vi "Rasnik_save.vi"() -> ()   [LabVIEW 2015]
uses:
  GlobalPath.vi
  Desktop/Mari/GlobalData.vi
panel:
  out "Script":path
  out "Logfile Path":path
  out "Filename selected":path
  out "standard output":string
  out "Y D10":dbl format="%.2f"
  out "Y D9":dbl format="%.2f"
  out "Y D8":dbl format="%.2f"
  out "Y D7":dbl format="%.2f"
  out "Y D6":dbl format="%.2f"
  out "Y D5":dbl format="%.2f"
  out "Y D4":dbl format="%.2f"
  out "Y D3":dbl format="%.2f"
  out "Y D2":dbl format="%.2f"
  out "Y D1":dbl format="%.2f"
  out "X D10":dbl format="%.2f"
  out "X D9":dbl format="%.2f"
  out "X D8":dbl format="%.2f"
  out "X D7":dbl format="%.2f"
  out "X D6":dbl format="%.2f"
  out "X D5":dbl format="%.2f"
  out "X D4":dbl format="%.2f"
  out "X D3":dbl format="%.2f"
  out "X D2":dbl format="%.2f"
  out "X D1":dbl format="%.2f"
  out "Latest file: 2":path
  out "y 6":string
  out "x 6":string
  in  "Done?":bool
  out "y 10":string
  out "x 10":string
  out "y 9":string
  out "x 9":string
  out "y 8":string
  out "x 8":string
  out "y 7":string
  out "x 7":string
  out "y 5":string
  out "x 5":string
  out "y 4":string
  out "x 4":string
  out "y 3":string
  out "x 3":string
  out "y 2":string
  out "x 2":string
  out "y 1":string
  out "x 1":string
  out "Lines":string[](array[string])
  out "Latest file:":path
  in  "Open Program":bool
  in  "c-ccd 3":bool caption="Setup the electronics for the C-CCD reading:\n- make sure the ethernet cables are connected on the minimal heads\n- check that the cable connecting the driver with the mux is plugged in\n- verify that the driver is on and connected to the LAN"
  in  "c-ccd":bool caption="Read the data file"
  # "Rasmask reading from PCBs on stiffback/table"
  # "Run the C-CCD reading program \n(the 10 Rasmasks are automatically read and the data saved)"
  # "Data file reading"
  # "The most recent data file created by the C-CCD program will be opened.\nOnce the \"read data file\" is clicked, the raw data and displacement should appear on the PCB schematics on the bottom."
  # "Displacement (um):"
  # "Raw Data (um):"
  # "Rasmask 1"
  # "Rasmask 2"
  # "Rasmask 1"
  # "Rasmask 2"
  # "Rasmask 3"
  # "Rasmask 4"
  # "Rasmask 3"
  # "Rasmask 4"
  # "Rasmask 6"
  # "Rasmask 5"
  # "Rasmask 6"
  # "Rasmask 5"
  # "Rasmask 7"
  # "Rasmask 8"
  # "Rasmask 7"
  # "Rasmask 8"
  # "Rasmask 9"
  # "Rasmask 10"
  # "Rasmask 9"
  # "Rasmask 10"
  # "Open the DB and load the Rarnik raw file:\nClick on the tab \"RO measurement\" and on the bottom click on \"Load Rasnik 1\" for the table and \"Load  Rasnik 2\" for the stiffback\nLoad the file that appears here --------------------------------------------------------------->\nPress \"SAve info to database\""
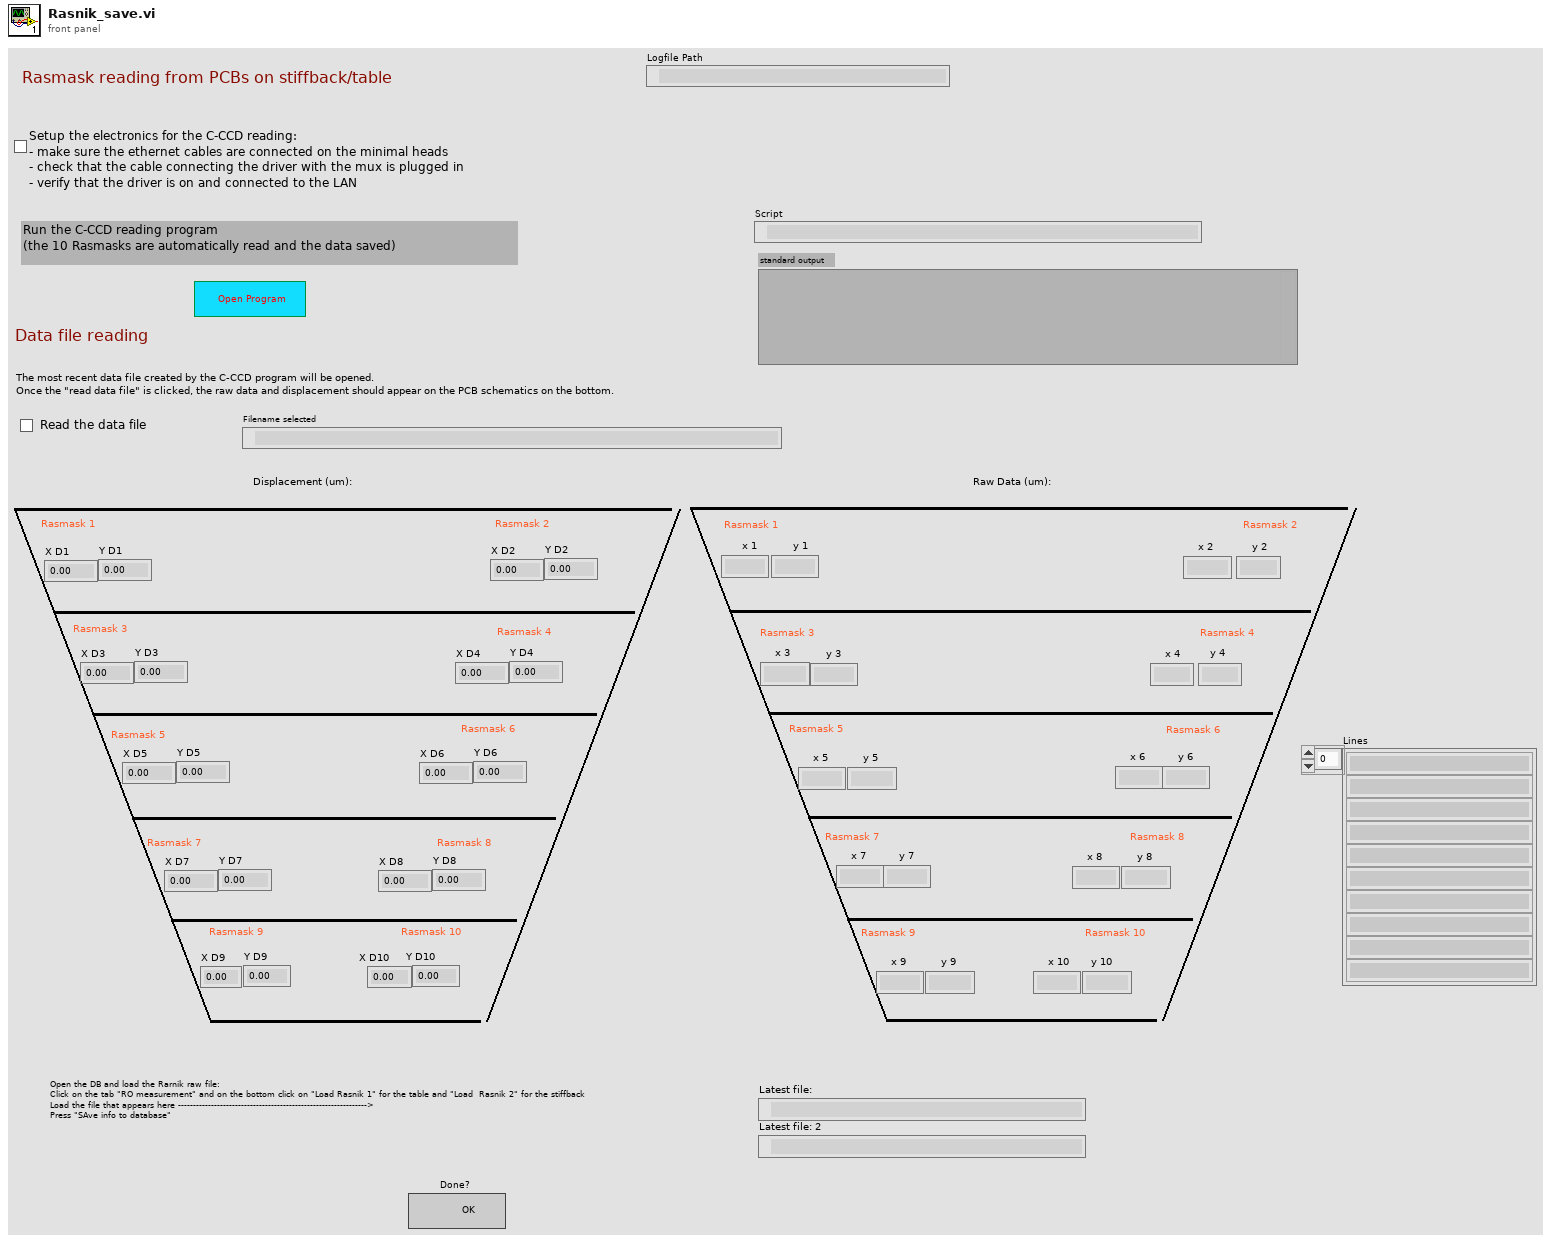
[diagram p1: front panel]
types:
  T1 = enum16{"open", "replace", "create", "open or create", "replace or create", "replace or create with confirmation"}
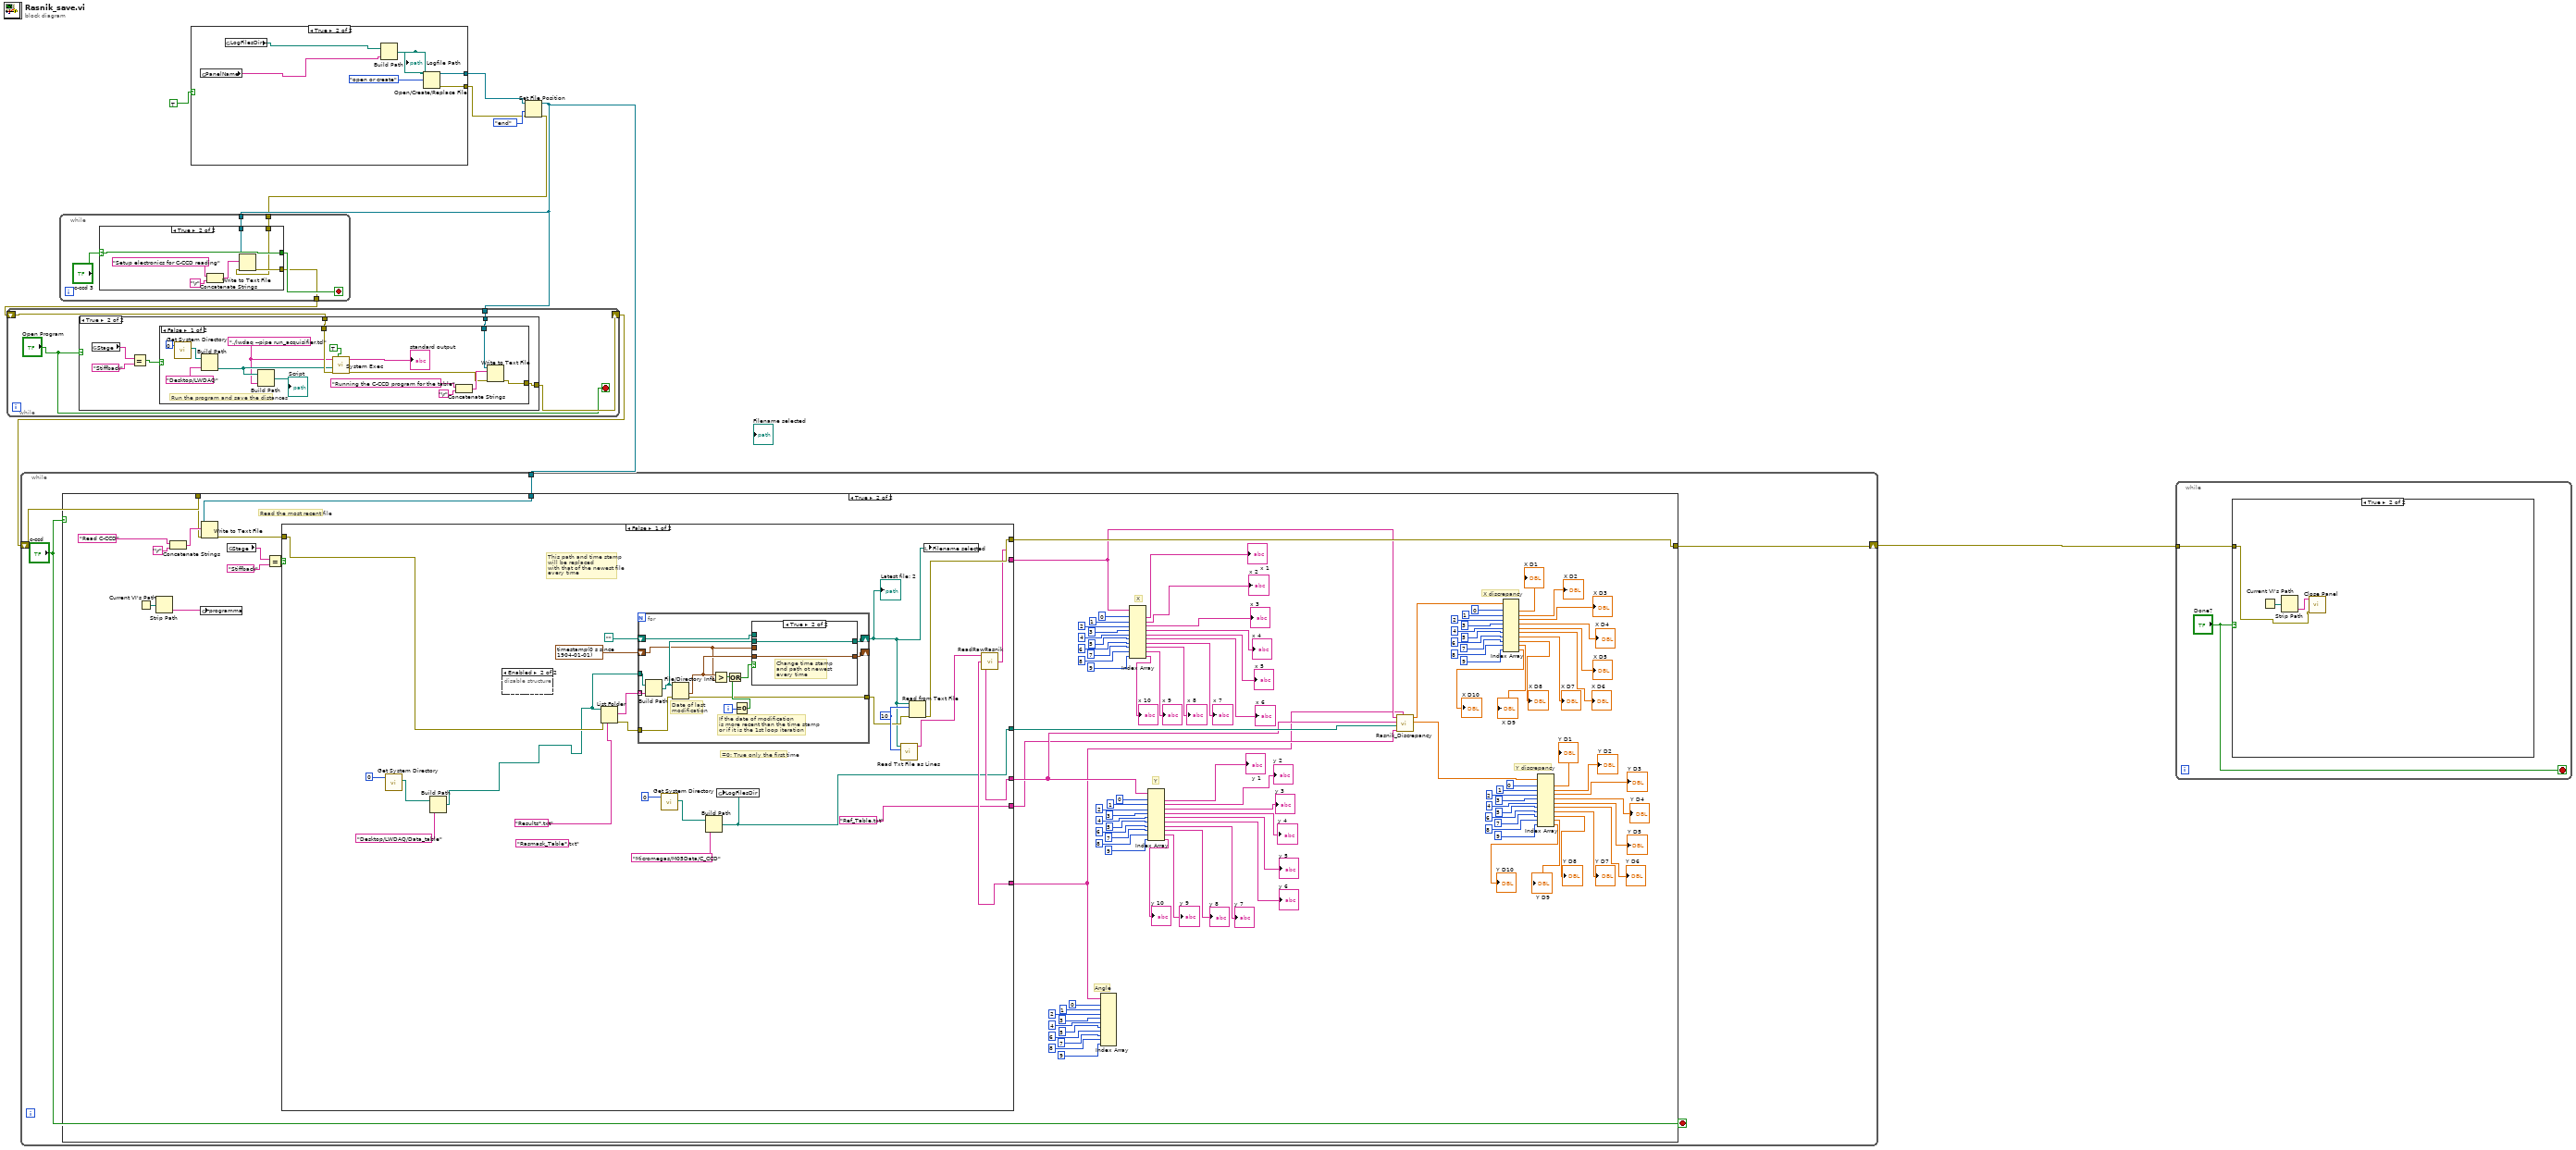
[diagram p0: block diagram]
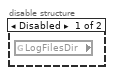
[diagram p4: hidden frame]
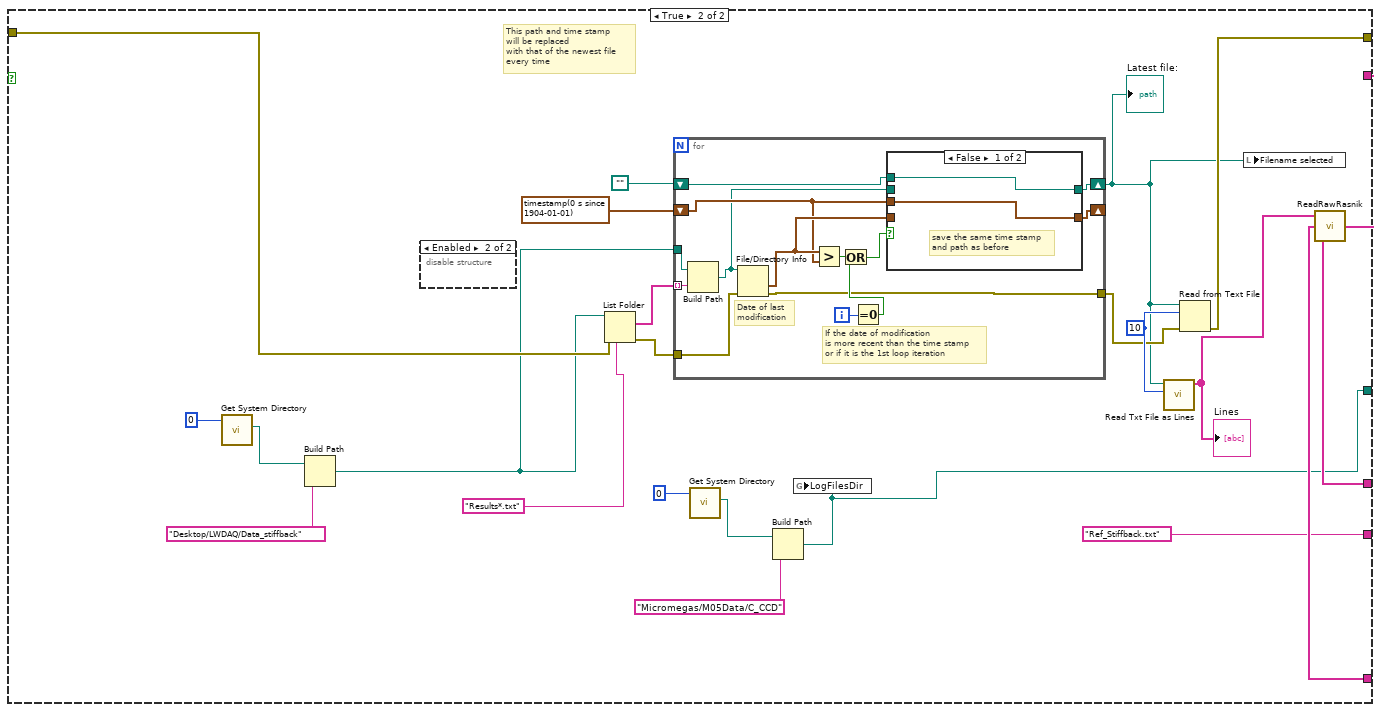
[diagram p6: hidden frame]
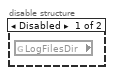
[diagram p7: hidden frame]
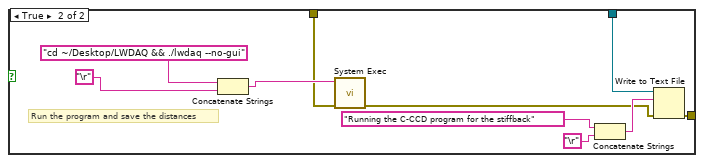
[diagram p11: hidden frame]
diagram:
  n1 = case shown="True" TRUE {
    tunnel: [_ w14] -> w3
    tunnel: [_ w13] -> w4
    frame False {
    }
    frame True {
      n2 = global read "GlobalData.vi" "PanelName"() -> (w10:string)
      n3 = global read "GlobalPath.vi" "LogFilesDir"() -> (w11:path)
      n4 = Build Path(base path=w11, name or relative path=w10) -> (appended path=w15:path)
      "Logfile Path" <- w15
      n5 = Open/Create/Replace File(file path (use dialog)=w15, operation (0:open)=T1."open or create") -> (refnum out=w14:refnum<file>, error out=w13:errorcluster)  [unwired: 4 in, 1 out]
    }
  }
  n6 = Set File Position(refnum=w3, from (0:start)=enum16{"start", "end", "current"}."end", error in=w4) -> (refnum out=w2:refnum<file>, error out=w1:errorcluster)  [unwired: 1 in]
  n7 = while {
    tunnel: w2 -> [w19]
    tunnel: [w17] -> w7
    tunnel: w1 -> [w16]
    stop <- w18 stop-if-true
    n8 = case shown="True" "c-ccd 3" {
      selector: "c-ccd 3" -> [_ w23]
      tunnel: [_ w24] -> w17
      tunnel: w19 -> [_ w21]
      tunnel: [_ w23] -> w18
      tunnel: w16 -> [_ w22]
      frame False {
      }
      frame True {
        n9 = Concatenate Strings("Setup electronics for C-CCD reading", "\r") -> (w27:string)
        n10 = Write to Text File(file (use dialog)=w21, text=w27, error in=w22) -> (error out=w24:errorcluster)  [unwired: 1 in, 2 out]
      }
    }
  }
  n11 = while {
    tunnel: w2 -> [w29]
    shift-right: [w30] -> w9
    shift-left: w7 -> [w31]
    stop <- "Open Program" stop-if-true
    n12 = case shown="True" "Open Program" {
      tunnel: w31 -> [w32 w35]
      tunnel: [w32 w34] -> w30
      tunnel: w29 -> [_ w33]
      frame False {
      }
      frame True {
        n13 = global read "GlobalData.vi" "Stage"() -> (w37:string)
        n14 = Equal?(x=w37, y="Stiffback") -> (x = y?=w36:bool)
        n15 = case shown="False" w36 {
          tunnel: w35 -> [w50 w57]
          tunnel: [w48 w55] -> w34
          tunnel: w33 -> [w47 w54]
          frame False {
            w40 = "./lwdaq --pipe run_acquisifier.tcl"
            # "Run the program and save the distances"
            n16 = call <vilib>:"Get System Directory.vi"("system directory type"=0) -> ("system directory"=w45:path)  [unwired: 10 in]
            n17 = Build Path(base path=w45, name or relative path="Desktop/LWDAQ") -> (appended path=w41:path)
            n18 = Build Path(base path=w41, name or relative path=w40) -> (appended path=→"Script":path)
            n19 = call <vilib>:"System Exec.vi"("wait until completion? (T)"=TRUE, "error in (no error)"=w50, "working directory"=w41, "command line"=w40) -> ("error out"=w49:errorcluster, "standard output"=→"standard output":string)  [unwired: 4 in, 2 out]
            n20 = Concatenate Strings("Running the C-CCD program for the table", "\r") -> (w53:string)
            n21 = Write to Text File(file (use dialog)=w47, text=w53, error in=w49) -> (error out=w48:errorcluster)  [unwired: 1 in, 2 out]
          }
          frame True {
            # "Run the program and save the distances"
            n22 = Concatenate Strings("cd ~/Desktop/LWDAQ && ./lwdaq --no-gui", "\r") -> (w62:string)
            n23 = call <vilib>:"System Exec.vi"("error in (no error)"=w57, "command line"=w62) -> ("error out"=w56:errorcluster)  [unwired: 6 in, 3 out]
            n24 = Concatenate Strings("Running the C-CCD program for the stiffback", "\r") -> (w60:string)
            n25 = Write to Text File(file (use dialog)=w54, text=w60, error in=w56) -> (error out=w55:errorcluster)  [unwired: 1 in, 2 out]
          }
        }
      }
    }
  }
  n26 = while {
    tunnel: w2 -> [w65]
    shift-right: [w66] -> w8
    shift-left: w9 -> [w67]
    stop <- "c-ccd" stop-if-true
    n27 = case shown="True" "c-ccd" {
      tunnel: w67 -> [w68 w169]
      tunnel: [w68 w167] -> w66
      tunnel: w65 -> [_ w166]
      frame False {
      }
      frame True {
        # "Y discrepancy"
        # "X discrepancy"
        # "Angle"
        # "Y"
        # "X"
        # "Read the most recent file"
        n28 = Current VI's Path() -> (path=w170:path)
        n29 = Strip Path(path=w170) -> (name=w171:string)  [unwired: 1 out]
        n30 = Concatenate Strings("Read C-CCD", "\r") -> (w177:string)
        n31 = global write "GlobalData.vi" "programma"(w171) -> ()
        n32 = Write to Text File(file (use dialog)=w166, text=w177, error in=w169) -> (error out=w168:errorcluster)  [unwired: 1 in, 2 out]
        n33 = global read "GlobalData.vi" "Stage"() -> (w173:string)
        n34 = Equal?(x=w173, y="Stiffback") -> (x = y?=w172:bool)
        n35 = case shown="False" w172 {
          tunnel: w168 -> [w189 w238]
          tunnel: [w192 w233] -> w167
          tunnel: [w191 w232] -> w114
          tunnel: [w193 w231] -> w113
          tunnel: [w190 w230] -> w69
          tunnel: [w179 w220] -> w115
          tunnel: ["Ref_Table.txt" "Ref_Stiffback.txt"] -> w112
          frame False {
            (unwired) "Rasmask_Table*.txt"
            w198 = 10
            # "=0: True only the first time"
            # "This path and time stamp\nwill be replaced\nwith that of the newest file \nevery time"
            n36 = call <vilib>:"Get System Directory.vi"("system directory type"=0) -> ("system directory"=w185:path)  [unwired: 10 in]
            n37 = Build Path(base path=w185, name or relative path="Desktop/LWDAQ/Data_table") -> (appended path=w184:path)
            n38 = disable-structure shown="Enabled" {
              frame Disabled {
                n39 = global read "GlobalPath.vi" "LogFilesDir"() -> ()  [unwired: 1 out]
              }
              frame Enabled {
              }
            }
            n40 = List Folder(path=w184, pattern="Results*.txt", error in=w189) -> (filenames=w194:string[], error out=w197:errorcluster)  [unwired: 1 in, 2 out]
            n41 = for {
              tunnel: w194 -> [w206] mode=indexing
              tunnel: w184 -> [w214]
              shift-right: [w210] -> _
              shift-left: timestamp(0 s since 1904-01-01) ("last mod 2") -> [w201]
              shift-right: [w209] -> w178
              shift-left: path "" -> [w207]
              tunnel: w197 -> [w204]
              tunnel: [w203] -> w196
              i -> [w212]
              # "If the date of modification\nis more recent than the time stamp\nor if it is the 1st loop iteration"
              # "Date of last\nmodification"
              n42 = Build Path(base path=w214, name or relative path=w206) -> (appended path=w205:path)
              n43 = File/Directory Info(path=w205, error in=w204) -> (last mod=w202:timestamp, error out=w203:errorcluster)  [unwired: 5 out]
              n44 = Greater?(x=w202, y=w201) -> (0:w213:bool)
              n45 = Equal To 0?(x=w212) -> (x = 0?=w211:bool)
              n46 = Or(x=w213, y=w211) -> (x .or. y?=w208:bool)
              n47 = case shown="True" w208 {
                tunnel: w201 -> [w216 _]
                tunnel: w202 -> [_ w218]
                tunnel: w205 -> [_ w217]
                tunnel: [w215 w217] -> w209
                tunnel: w207 -> [w215 _]
                tunnel: [w216 w218] -> w210
                frame False {
                  # "save the same time stamp \nand path as before"
                }
                frame True {
                  # "Change time stamp\nand path ot newest \nevery time"
                }
              }
            }
            "Latest file: 2" <- w178
            n48 = call <vilib>:"Get System Directory.vi"("system directory type"=0) -> ("system directory"=w181:path)  [unwired: 10 in]
            n49 = Build Path(base path=w181, name or relative path="Micromegas/M05Data/C_CCD") -> (appended path=w179:path)
            n50 = global write "GlobalPath.vi" "LogFilesDir"(w179) -> ()
            n51 = call "Read Txt File as Lines.vi"("Lines to Read"=w198, "file path (use dialog)"=w178) -> ("Lines"=w195:string[])  [unwired: 8 in, 1 out]
            n52 = Read from Text File(file (use dialog)=w178, count=w198, error in=w196) -> (error out=w192:errorcluster)  [unwired: 1 in, 3 out]
            n53 = local write "Filename selected"(w178) -> ()
            n54 = call "ReadRawRasnik.vi"("Lines"=w195) -> ("X cluster"=w191:string[], "Y cluster"=w193:string[], "angle cluster"=w190:string[])
          }
          frame True {
            w239 = 10
            # "This path and time stamp\nwill be replaced\nwith that of the newest file \nevery time"
            n55 = call <vilib>:"Get System Directory.vi"("system directory type"=0) -> ("system directory"=w227:path)  [unwired: 10 in]
            n56 = Build Path(base path=w227, name or relative path="Desktop/LWDAQ/Data_stiffback") -> (appended path=w221:path)
            n57 = disable-structure shown="Enabled" {
              frame Disabled {
                n58 = global read "GlobalPath.vi" "LogFilesDir"() -> ()  [unwired: 1 out]
              }
              frame Enabled {
              }
            }
            n59 = List Folder(path=w221, pattern="Results*.txt", error in=w238) -> (filenames=w234:string[], error out=w237:errorcluster)  [unwired: 1 in, 2 out]
            n60 = for {
              tunnel: w234 -> [w245] mode=indexing
              tunnel: w221 -> [w255]
              shift-right: [w250] -> _
              shift-left: timestamp(0 s since 1904-01-01) ("last mod 2") -> [w248]
              shift-right: [w249] -> w219
              shift-left: path "" -> [w246]
              tunnel: w237 -> [w243]
              tunnel: [w242] -> w236
              i -> [w253]
              # "If the date of modification\nis more recent than the time stamp\nor if it is the 1st loop iteration"
              # "Date of last\nmodification"
              n61 = Build Path(base path=w255, name or relative path=w245) -> (appended path=w244:path)
              n62 = File/Directory Info(path=w244, error in=w243) -> (last mod=w251:timestamp, error out=w242:errorcluster)  [unwired: 5 out]
              n63 = Greater?(x=w251, y=w248) -> (0:w254:bool)
              n64 = Equal To 0?(x=w253) -> (x = 0?=w252:bool)
              n65 = Or(x=w254, y=w252) -> (x .or. y?=w247:bool)
              n66 = case shown="False" w247 {
                tunnel: w248 -> [w257 _]
                tunnel: w251 -> [_ w259]
                tunnel: w244 -> [_ w258]
                tunnel: [w256 w258] -> w249
                tunnel: w246 -> [w256 _]
                tunnel: [w257 w259] -> w250
                frame False {
                  # "save the same time stamp \nand path as before"
                }
                frame True {
                  # "Change time stamp\nand path ot newest \nevery time"
                }
              }
            }
            "Latest file:" <- w219
            n67 = call <vilib>:"Get System Directory.vi"("system directory type"=0) -> ("system directory"=w223:path)  [unwired: 10 in]
            n68 = Build Path(base path=w223, name or relative path="Micromegas/M05Data/C_CCD") -> (appended path=w220:path)
            n69 = global write "GlobalPath.vi" "LogFilesDir"(w220) -> ()
            n70 = call "Read Txt File as Lines.vi"("Lines to Read"=w239, "file path (use dialog)"=w219) -> ("Lines"=w235:string[])  [unwired: 8 in, 1 out]
            "Lines" <- w235
            n71 = Read from Text File(file (use dialog)=w219, count=w239, error in=w236) -> (error out=w233:errorcluster)  [unwired: 1 in, 3 out]
            n72 = local write "Filename selected"(w219) -> ()
            n73 = call "ReadRawRasnik.vi"("Lines"=w235) -> ("X cluster"=w232:string[], "Y cluster"=w231:string[], "angle cluster"=w230:string[])
          }
        }
        n74 = Index Array(array=w69, index #1=0, index #2=1, index #3=2, index #4=3, index #5=4, index #6=5, index #7=6, index #8=7, index #9=8, index #10=9) -> ()  [unwired: 10 out]
        n75 = Index Array(array=w114, index #1=0, index #2=1, index #3=2, index #4=3, index #5=4, index #6=5, index #7=6, index #8=7, index #9=8, index #10=9) -> (element #1=→"x 1":string, element #2=→"x 2":string, element #3=→"x 3":string, element #4=→"x 4":string, element #5=→"x 5":string, element #6=→"x 6":string, element #7=→"x 7":string, element #8=→"x 8":string, element #9=→"x 9":string, element #10=→"x 10":string)
        n76 = Index Array(array=w113, index #1=0, index #2=1, index #3=2, index #4=3, index #5=4, index #6=5, index #7=6, index #8=7, index #9=8, index #10=9) -> (element #1=→"y 1":string, element #2=→"y 2":string, element #3=→"y 3":string, element #4=→"y 4":string, element #5=→"y 5":string, element #6=→"y 6":string, element #7=→"y 7":string, element #8=→"y 8":string, element #9=→"y 9":string, element #10=→"y 10":string)
        n77 = call "Rasnik_Discrepancy.vi"("angle array"=w69, "pattern"=w112, "path"=w115, "Y array"=w113, "X array"=w114) -> ("Y discrepancy"=w71:dbl[], "X discrepancy"=w70:dbl[])  [unwired: 4 in, 1 out]
        n78 = Index Array(array=w70, index #1=0, index #2=1, index #3=2, index #4=3, index #5=4, index #6=5, index #7=6, index #8=7, index #9=8, index #10=9) -> (element #1=→"X D1":dbl, element #2=→"X D2":dbl, element #3=→"X D3":dbl, element #4=→"X D4":dbl, element #5=→"X D5":dbl, element #6=→"X D6":dbl, element #7=→"X D7":dbl, element #8=→"X D8":dbl, element #9=→"X D9":dbl, element #10=→"X D10":dbl)
        n79 = Index Array(array=w71, index #1=0, index #2=1, index #3=2, index #4=3, index #5=4, index #6=5, index #7=6, index #8=7, index #9=8, index #10=9) -> (element #1=→"Y D1":dbl, element #2=→"Y D2":dbl, element #3=→"Y D3":dbl, element #4=→"Y D4":dbl, element #5=→"Y D5":dbl, element #6=→"Y D6":dbl, element #7=→"Y D7":dbl, element #8=→"Y D8":dbl, element #9=→"Y D9":dbl, element #10=→"Y D10":dbl)
      }
    }
  }
  n80 = while {
    tunnel: w8 -> [w261]
    stop <- "Done?" stop-if-true
    n81 = case shown="True" "Done?" {
      tunnel: w261 -> [_ w262]
      frame False {
      }
      frame True {
        n82 = Current VI's Path() -> (path=w263:path)
        n83 = Strip Path(path=w263) -> (name=w264:string)  [unwired: 1 out]
        n84 = call <vilib>:"Close Panel.vi"("error in (no error)"=w262, "VI name"=w264) -> ()  [unwired: 9 in, 1 out]
      }
    }
  }
